vi "ConnectUnflattenFromJSONNode.vi"(0 "VI Ref In":refnum<vi>, 5 "Control Terminal References":T1[](array[typedef]), 11 "Error In":errorcluster) -> (15 "Error Out":errorcluster)   [LabVIEW 2019, in "JsonToCluster.lvlib"]
doc: "This VI connects Unflatten from JSON node with its equivalent control terminals"
uses:
  JsonToCluster.lvlib
  _Controls/ControlTerminalReference.ctl
  <vilib>/SLL Drona/APIs/Get/GetControlRef/GetControlRefByPath.vi
  <vilib>/SLL Drona/Drona.lvlib
  <vilib>/SLL Drona/APIs/Get/GetControlRef/GetControlRef.lvlib
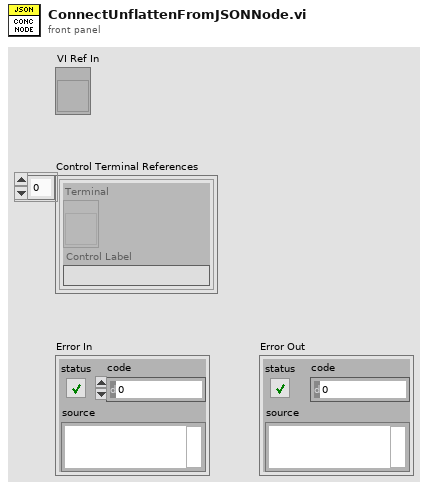
[diagram p1: front panel]
types:
  T1 = typedef "JsonToCluster.lvlib/ControlTerminalReference.ctl" = cluster{"Terminal":refnum<vi>, "Control Label":string}
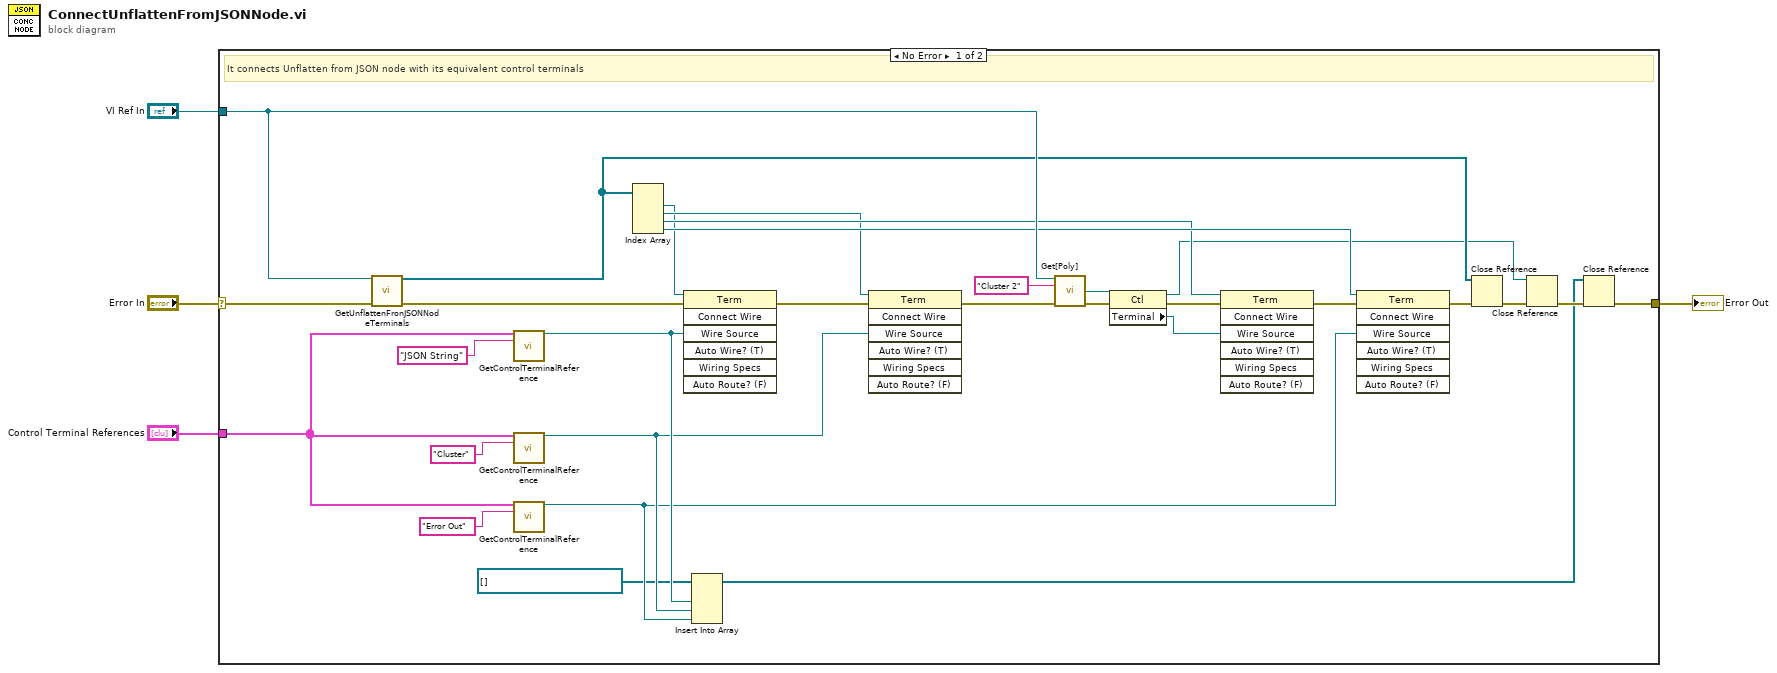
[diagram p0: block diagram]
diagram:
  n1 = case shown="No Error" "Error In" {
    selector: "Error In" -> [w16 w35]
    tunnel: "Control Terminal References" -> [w33 _]
    tunnel: "VI Ref In" -> [w27 _]
    tunnel: [w10 w35] -> w2
    frame No Error {
      # "It connects Unflatten from JSON node with its equivalent control terminals"
      n2 = call "GetUnflattenFronJSONNodeTerminals.vi"("VI Ref In"=w27, "Error In"=w16) -> ("Node Terminal References"=w14:refnum<vi>[], "Error Out"=w18:errorcluster)  [unwired: 12 in]
      n3 = call "GetControlTerminalReference.vi"("Control Terminal References"=w33, "Control Name"="JSON String" ("y")) -> ("Terminal Reference"=w9:refnum<vi>)  [unwired: 13 in]
      n4 = call "GetControlTerminalReference.vi"("Control Terminal References"=w33, "Control Name"="Cluster") -> ("Terminal Reference"=w8:refnum<vi>)  [unwired: 13 in]
      n5 = call "GetControlTerminalReference.vi"("Control Terminal References"=w33, "Control Name"="Error Out") -> ("Terminal Reference"=w7:refnum<vi>)  [unwired: 13 in]
      n6 = Index Array(array=w14) -> (element #1=w17:refnum<vi>, element #2=w20:refnum<vi>, element #3=w21:refnum<vi>, element #4=w25:refnum<vi>)  [unwired: 4 in]
      n7 = invoke class="Term" method="Connect Wire"(reference=w17, error in=w18, "Wire Source"=w9) -> (error out=w19:errorcluster)  [unwired: 4 in, 6 out]
      n8 = Insert Into Array(array=refnum<vi>[] [], new element #1=w9, new element #2=w8, new element #3=w7) -> (w5:refnum<vi>[])  [unwired: 1 in]
      n9 = invoke class="Term" method="Connect Wire"(reference=w20, error in=w19, "Wire Source"=w8) -> (error out=w26:errorcluster)  [unwired: 4 in, 6 out]
      n10 = call-poly <vilib>:"Get[Poly].vi"("VI Reference In"=w27, "Control Path"="Cluster 2", "error In"=w26) -> ("Ctl Refnum"=w29:refnum<vi>, "error out"=w30:errorcluster)  [unwired: 10 in, 1 out]
      n11 = property class="Ctl"(reference=w29, error in=w30) -> (reference out=w13:refnum<vi>, error out=w22:errorcluster, "Terminal"=w23:refnum<vi>)
      n12 = invoke class="Term" method="Connect Wire"(reference=w21, error in=w22, "Wire Source"=w23) -> (error out=w24:errorcluster)  [unwired: 4 in, 6 out]
      n13 = invoke class="Term" method="Connect Wire"(reference=w25, error in=w24, "Wire Source"=w7) -> (error out=w15:errorcluster)  [unwired: 4 in, 6 out]
      n14 = Close Reference(reference=w14, error in (no error)=w15) -> (error out=w12:errorcluster)
      n15 = Close Reference(reference=w13, error in (no error)=w12) -> (error out=w11:errorcluster)
      n16 = Close Reference(reference=w5, error in (no error)=w11) -> (error out=w10:errorcluster)
    }
    frame Error {
      # "If error, this case pass that error message only"
    }
  }
  "Error Out" <- w2
